vi "OM Setup.vi"() -> ()   [LabVIEW 2009]
uses:
  lib/Data Access Objects/Metadata/LBCB Number.ctl
  lib/Data Access Objects/Metadata/LBCB Settings.ctl
  lib/Data Access Objects/Metadata/LBCB Size.ctl
  lib/Data Access Objects/Metadata/LBCB Type.ctl
  lib/Data Access Objects/Application/Number Of LBCBs.ctl
  lib/Data Access Objects/Metadata/LBCB Location.ctl
  lib/Data Access Objects/Metadata/Actuator Matrix.ctl
  lib/Data Access Objects/Metadata/Actuator Point.ctl
  lib/Data Access Objects/Metadata/Cartesian Matrix.ctl
  lib/Data Access Objects/Metadata/Cartesian Point.ctl
  lib/Data Access Objects/Autobalance/Autobalance Control Parameters.ctl
  lib/Data Access Objects/Application/App Parameters.ctl
  lib/Data Access Objects/Application/Timing Parameters.ctl
  lib/Data Access Objects/Metadata/LBCB Position.ctl
  lib/MixedMode/Stiffness Matrix.ctl
  lib/Data Access Objects/Metadata/Cartesian Force Vector.ctl
  lib/Data Access Objects/Limits/Limit Boundary Parameters.ctl
  Popups/External Sensor Specs.ctl
  lib/Data Access Objects/Metadata/Actuator Channel Names.ctl
  lib/MixedMode/Ramp Time Input.ctl
  lib/MixedMode/Ramp Control.ctl
  lib/Data Access Objects/Application/Network Parameters.ctl
  lib/Data Access Objects/Mixed Mode/Force Control Parameters.ctl
  Popups/Update Actions.ctl
  lib/Data Access Objects/Metadata/Persistant DAO Actions.ctl
panel:
  in  "Rigid Connection":bool
  in  "LBCB Number Button":bool
  in  "Number of LBCBs":T1
  in  "Save":bool
  in  "Load":bool
  in  "OM Setup Page Tab":T2(tab)
  in  "Act Disp Bnd":T3 caption="Actuator Disp Limit \nBoundary Parameters"
  in  "Actuator Force Limits":T4
  in  "Actuator Stroke Limits":T4
  in  "Command Voltage Limit":T4
  in  "Act Force Bnd":T3 caption="Actuator Force Limit \nBoundary Parameters"
  in  "Cartesian Displacement":T6
  in  "Cartesian Force Limit":T6
  in  "Cart Force Bnd":T3 caption="Cartesian Force Limit \nBoundary Parameters"
  in  "Cart Trans Bnd":T3 caption="Cartesian Translation Limit \nBoundary Parameters"
  in  "Cart Rot Bnd":T3 caption="Cartesian Rotation Limit \nBoundary Parameters"
  in  "Cart Mmt Bnd":T3 caption="Cartesian Moment Limit \nBoundary Parameters"
  in  "Auto Balance Control":T8={"Number of Samples"=0, "Delay After Cmd"=0, "Maximum Command"=0.0, "1/4 Linear Range"=0.5}
  in  "Auto Balance Error Window":T5
  in  "I Gain":T5
  in  "P Gain":T5
  in  "NTCP Network":T9={"Port Number"=0, "Notification Name"="DataAvailableForTransmission", "Wait For Notification Timeout"=1000}
  in  "DAQ Link Network":T9={"Port Number"=0, "Notification Name"="DataAvailableForTransmission", "Wait For Notification Timeout"=1000}
  in  "Application Timing and Logging":T10
  in  "LBCB Position":T12={"Motion Center"=[0.0, 0.0, 0.0], "Transformation Matrix"=[[1.0, 0.0, 0.0, 0.0, 0.0, 0.0], [0.0, 1.0, 0.0, 0.0, 0.0, 0.0], [0.0, 0.0, 1.0, 0.0, 0.0, 0.0], [0.0, 0.0, 0.0, 1.0, 0.0, 0.0], [0.0, 0.0, 0.0, 0.0, 1.0, 0.0], [0.0, 0.0, 0.0, 0.0, 0.0, 1.0]]}
  in  "LBCB Settings":T13={"Size"=enum."1/5th-scale LBCB", "Type"=enum."Left Hand Type"}
  in  "Force Control Parameters":T16
  in  "Stiffness Limit":T6
  in  "Force Group Priorities":T7
  in  "Default Ramp Times":T17
  in  "Force Error Range":T19
  in  "Jacobian Gain":T7
  in  "Max Increment":T7
  in  "Stiffness Jacobian":T20=[[1000000.0, 0.0, 0.0, 0.0, 0.0, 0.0], [0.0, 1000000.0, 0.0, 0.0, 0.0, 0.0], [0.0, 0.0, 1000000.0, 0.0, 0.0, 0.0], [0.0, 0.0, 0.0, 1000000.0, 0.0, 0.0], [0.0, 0.0, 0.0, 0.0, 1000000.0, 0.0], [0.0, 0.0, 0.0, 0.0, 0.0, 1000000.0]]
  in  "Servo Error Offset":T5
  in  "LVDT  Offset":T5
  in  "Load Cell  Offset":T5
  in  "Load Cell Sensitivity":T5
  in  "Command Sensitivity":T5
  in  "LVDT Sensitivity":T5
  in  "Command Channels":T21
  in  "LVDT Channels":T21
  in  "Load Cell Channels":T21
  in  "Servo Error  Channels":T21
  in  "External Sensor Specs":T22[](array[typedef])
  in  "OM  Location":T23
  in  "Ok":bool
  in  "LBCB Number":T24
  # "(Volts)"
  # "Interval is in Seconds\nRate is in Samples per Second"
  # "(inch)"
  # "X"
  # "(inch)"
  # "Y"
  # "(inch)"
  # "Z"
  # "Xglobal = T*Xlocal"
  # "DAQMx Global Channel"
  # "Display Name"
  # "Sensiitivity"
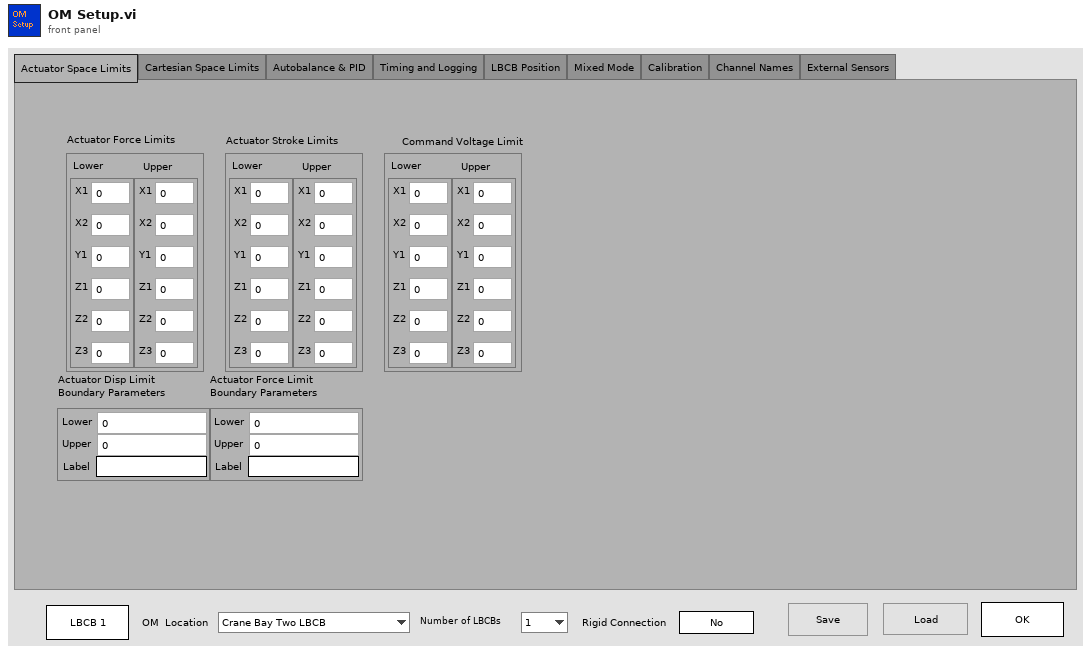
[diagram p1: front panel]
types:
  T1 = typedef "Number Of LBCBs.ctl" = enum16{"1", "2"}
  T2 = enum32{"Actuator Space Limits", "Cartesian Space Limits", "Autobalance & PID", "Timing and Logging", "LBCB Position", "Mixed Mode", "Calibration", "Channel Names", "External Sensors"}
  T3 = typedef "Limit Boundary Parameters.ctl" = cluster{"Lower":dbl, "Upper":dbl, "Label":string}
  T4 = typedef "Actuator Matrix.ctl" = cluster{"Lower":T5, "Upper":T5}
  T5 = typedef "Actuator Point.ctl" = cluster{"X1":dbl, "X2":dbl, "Y1":dbl, "Z1":dbl, "Z2":dbl, "Z3":dbl}
  T6 = typedef "Cartesian Matrix.ctl" = cluster{"Lower":T7, "Upper":T7}
  T7 = typedef "Cartesian Point.ctl" = cluster{"Dx":dbl, "Dy":dbl, "Dz":dbl, "Rx":dbl, "Ry":dbl, "Rz":dbl}
  T8 = typedef "Autobalance Control Parameters.ctl" = cluster{"Number of Samples":i32, "Delay After Cmd":i32, "Maximum Command":dbl, "1/4 Linear Range":dbl}
  T9 = typedef "Network Parameters.ctl" = cluster{"Port Number":u16, "Notification Name":string, "Wait For Notification Timeout":i32}
  T10 = typedef "App Parameters.ctl" = cluster{"Monitor Loop":T11, "Ramp Time":T11, "Log Loop":T11, "TCP to DAQ":T11, "Logging Directory":path, "Log File Size (MBytes)":i64, "Volt Logging Loop":T11}
  T11 = typedef "Timing Parameters.ctl" = cluster{"Interval":dbl, "Rate ":dbl}
  T12 = typedef "LBCB Position.ctl" = cluster{"Motion Center":dbl[], "Transformation Matrix":dbl[][]}
  T13 = typedef "LBCB Settings.ctl" = cluster{"Size":T14, "Type":T15}
  T14 = typedef "LBCB Size.ctl" = enum16{"1/5th-scale LBCB", "Full-scale LBCB", "Portable LBCB"}
  T15 = typedef "LBCB Type.ctl" = enum16{"Right Hand Type", "Left Hand Type"}
  T16 = typedef "Force Control Parameters.ctl" = cluster{"Use Force Error Range Ratios":bool, "Use Group Priorities":bool, "Multi Command Update":bool, "Use Tru Mixed Mode":bool}
  T17 = typedef "Ramp Time Input.ctl" = cluster{"Directional":T18, "Iterative":T18}
  T18 = typedef "Ramp Control.ctl" = cluster{"Ramp":dbl, "Stabilize":dbl, "Hold":dbl}
  T19 = typedef "Cartesian Force Vector.ctl" = cluster{"Fx":dbl, "Fy":dbl, "Fz":dbl, "Mx":dbl, "My":dbl, "Mz":dbl}
  T20 = typedef "Stiffness Matrix.ctl" = dbl[][]
  T21 = typedef "Actuator Channel Names.ctl" = cluster{"X1":refnum<k21>, "X2":refnum<k21>, "Y1":refnum<k21>, "Z1":refnum<k21>, "Z2":refnum<k21>, "Z3":refnum<k21>}
  T22 = typedef "External Sensor Specs.ctl" = cluster{"DAQmx Global Channel":refnum<k21>, "Display Name":string, "Sensitivity":dbl}
  T23 = typedef "LBCB Location.ctl" = enum16{"Crane Bay Two LBCB", "Crane Bay One LBCB", "5th Scale Two LBCB", "5th Scale One LBCB", "Portable LBCB"}
  T24 = typedef "LBCB Number.ctl" = enum16{"LBCB1", "LBCB2"}
  T25 = typedef "Update Actions.ctl" = enum16{"Update", "Exit"}
  T26 = typedef "Persistant DAO Actions.ctl" = enum16{"Init", "Get", "Set", "Load", "Save"}
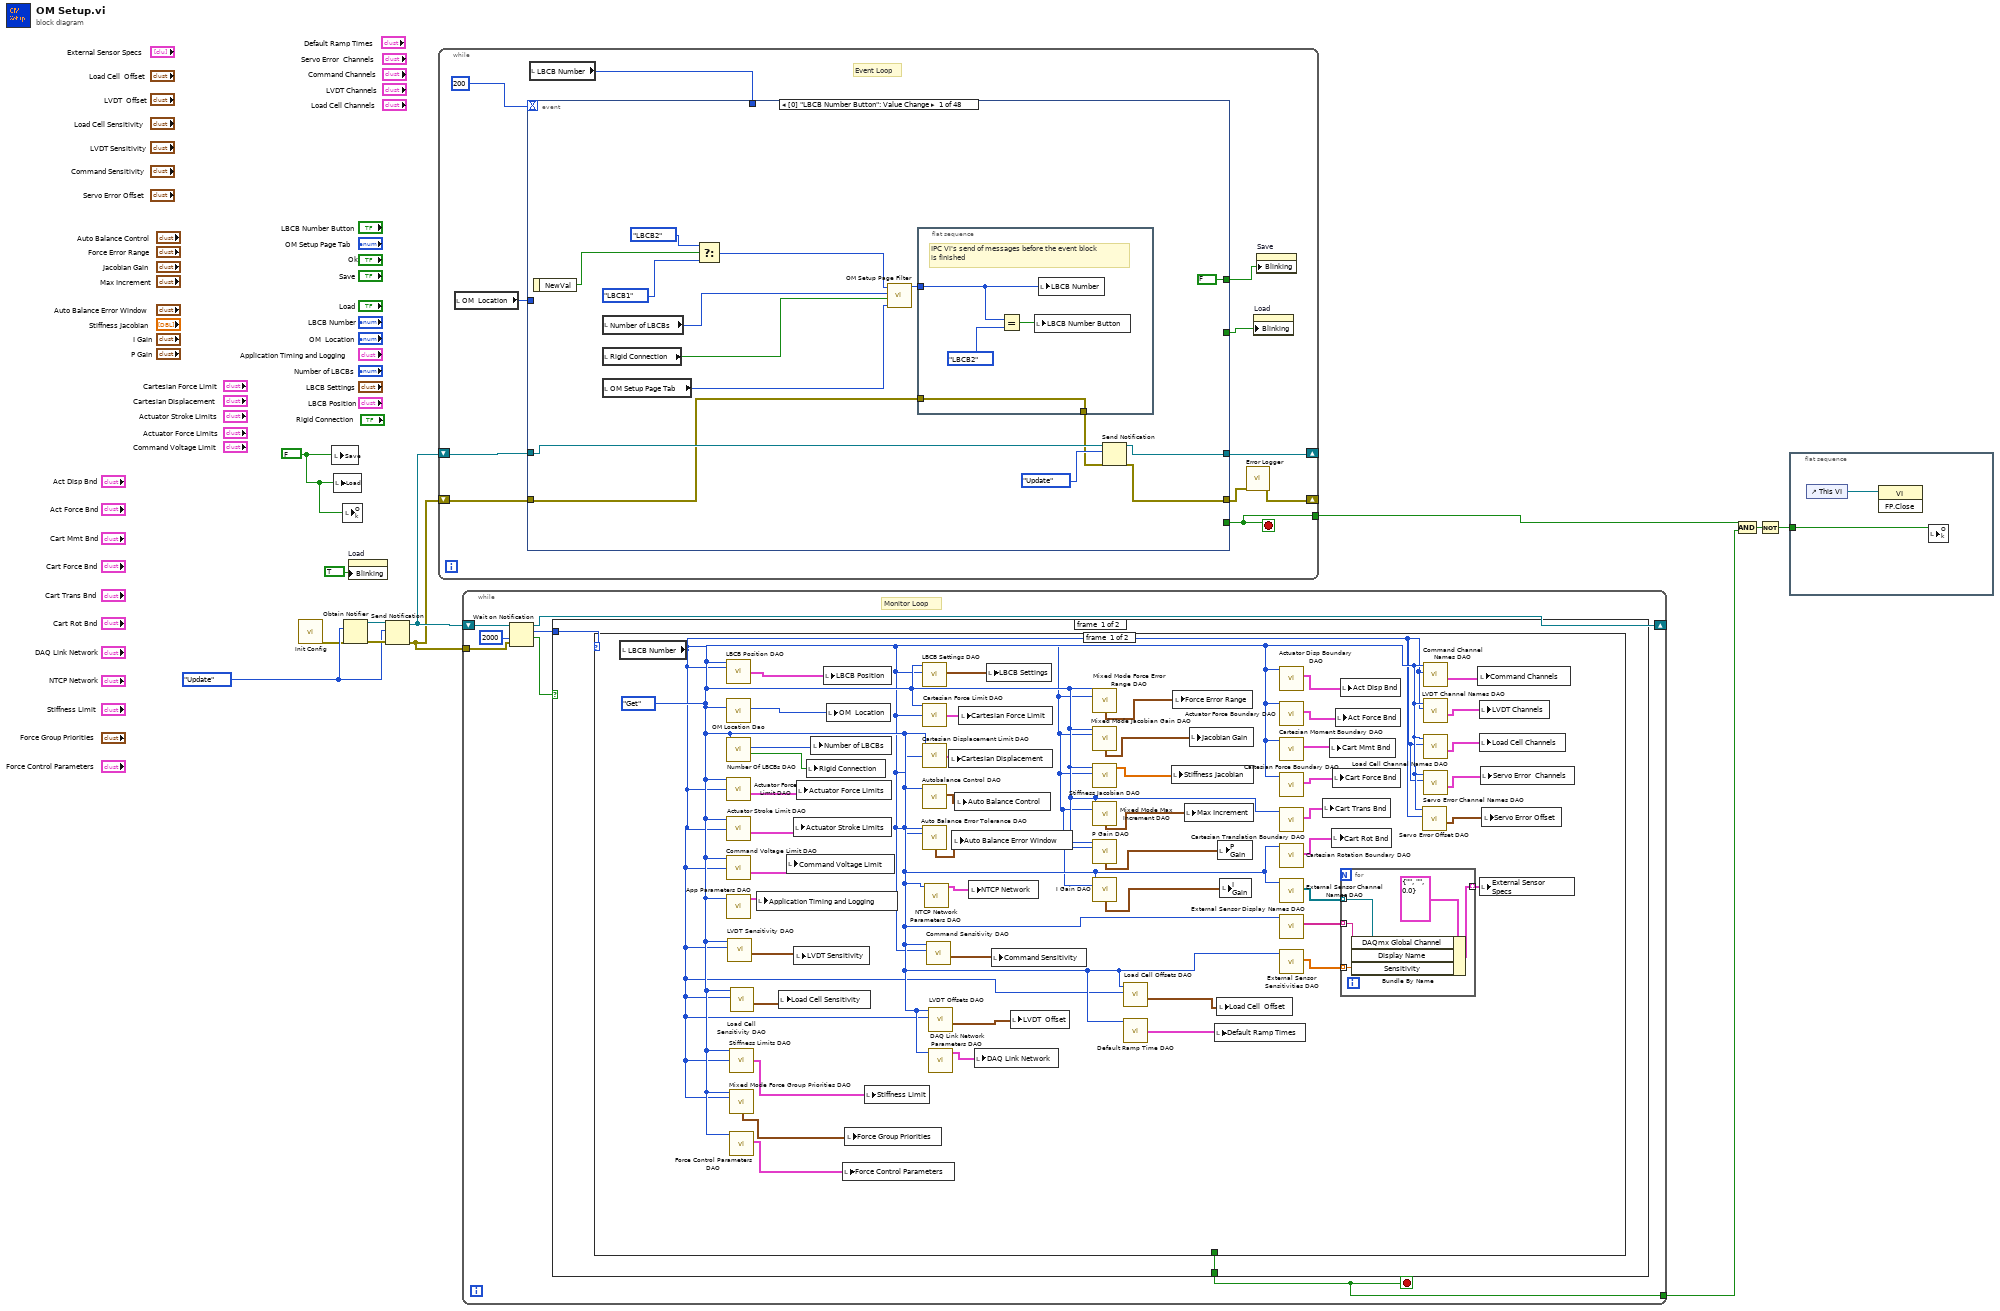
[diagram p0: block diagram]
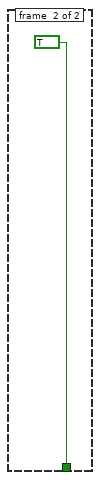
[diagram p2: hidden frame]
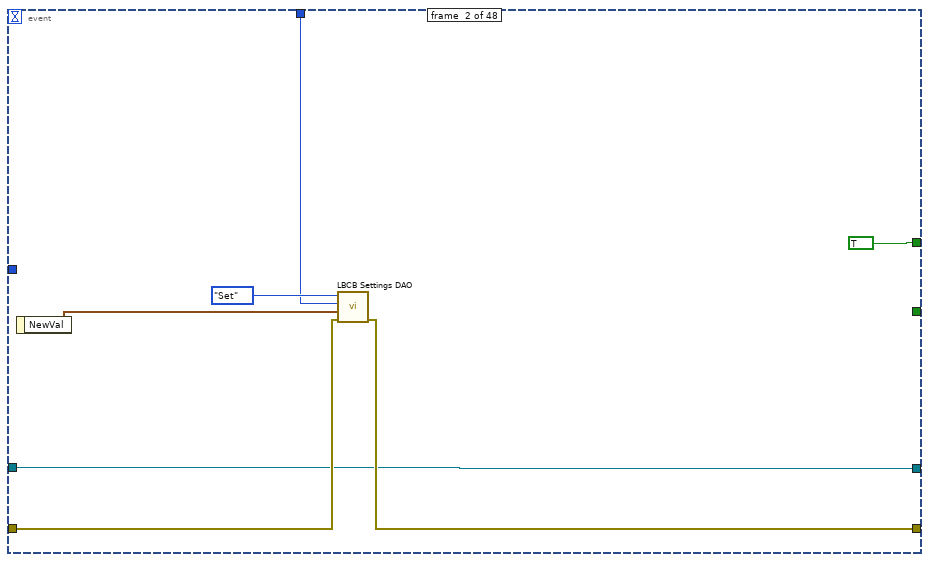
[diagram p4: hidden frame]
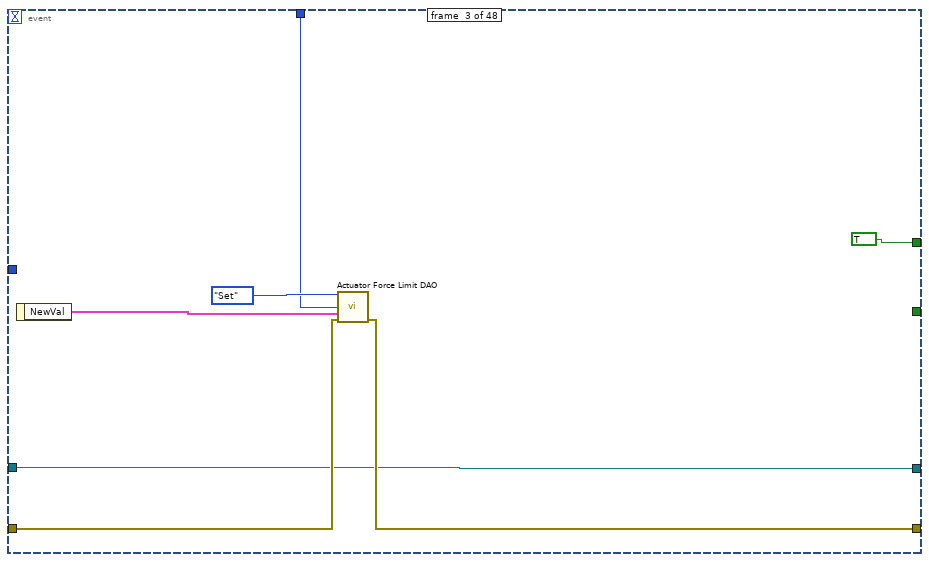
[diagram p5: hidden frame]
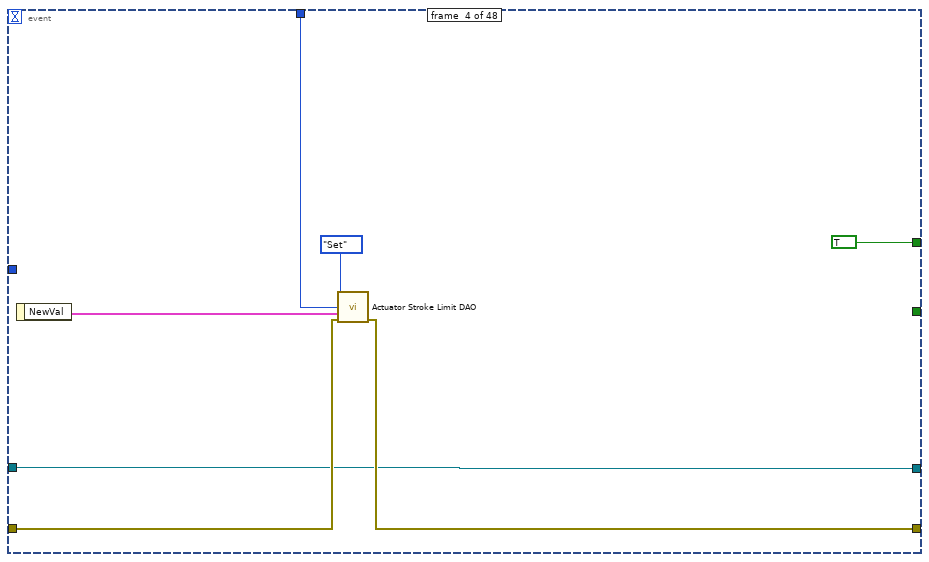
[diagram p6: hidden frame]
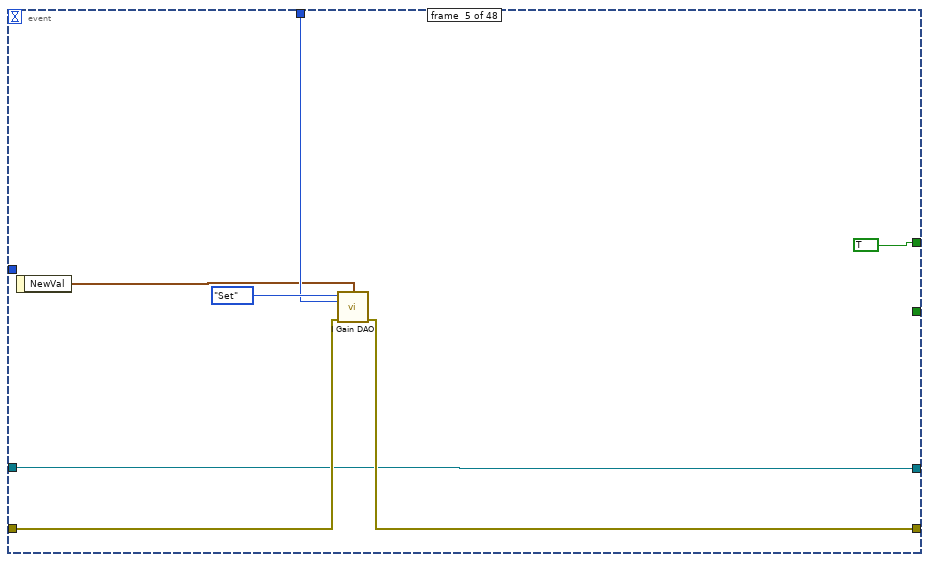
[diagram p7: hidden frame]
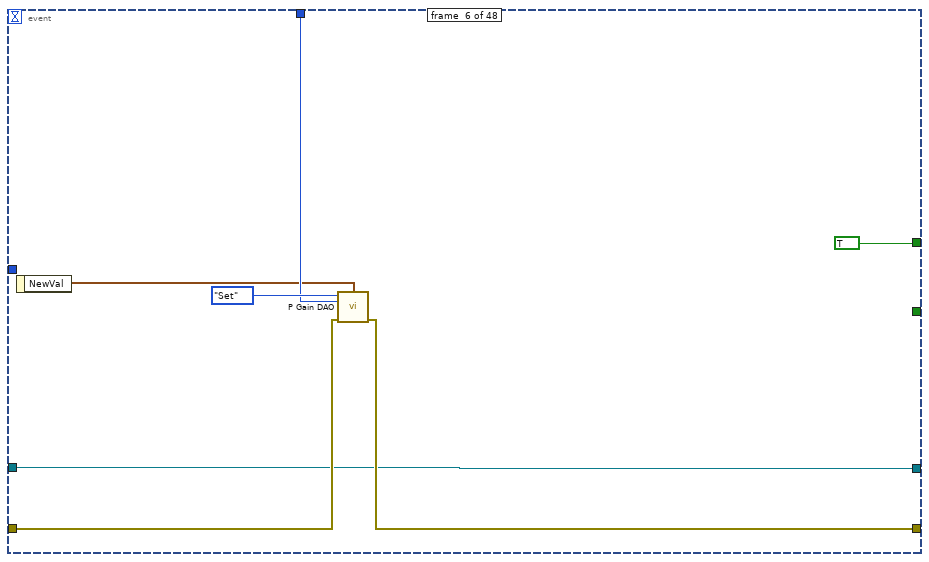
[diagram p8: hidden frame]
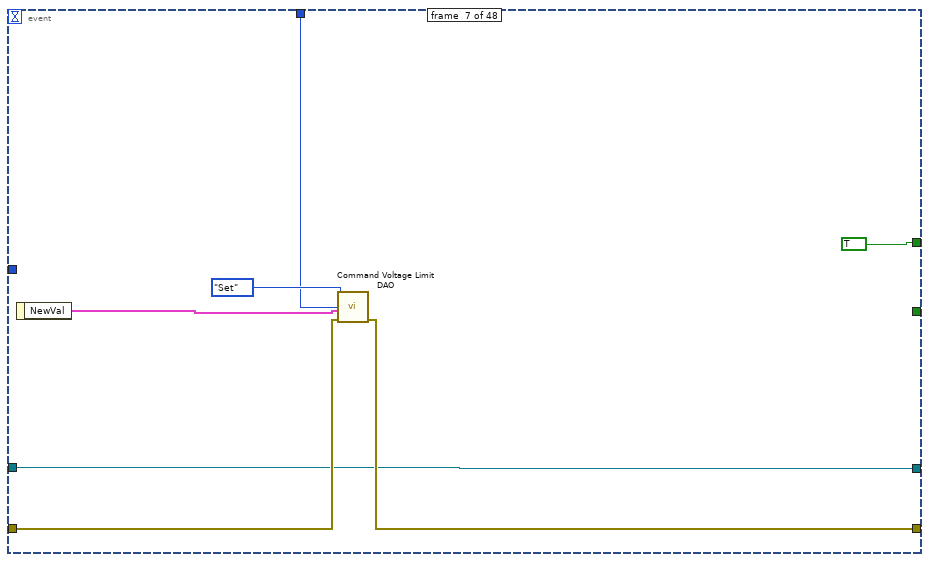
[diagram p9: hidden frame]
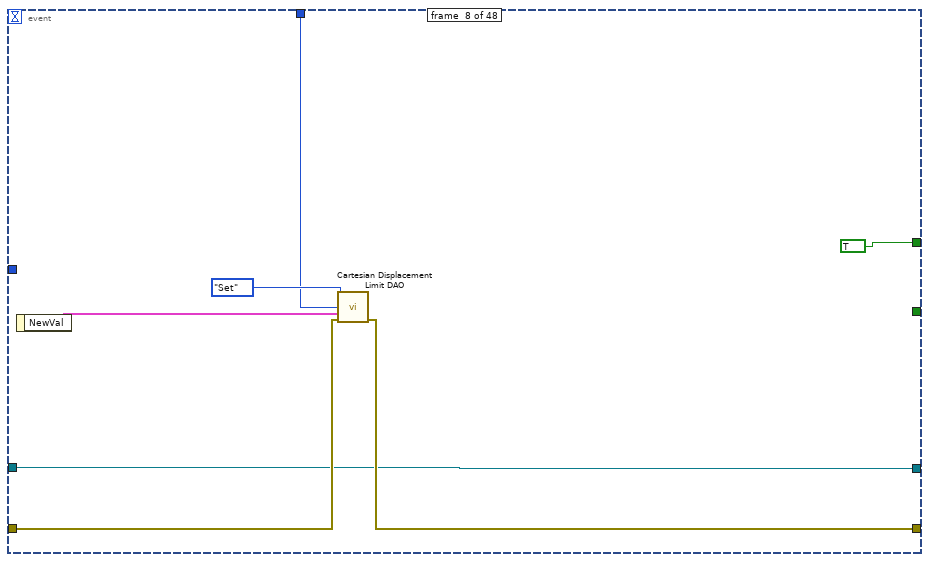
[diagram p10: hidden frame]
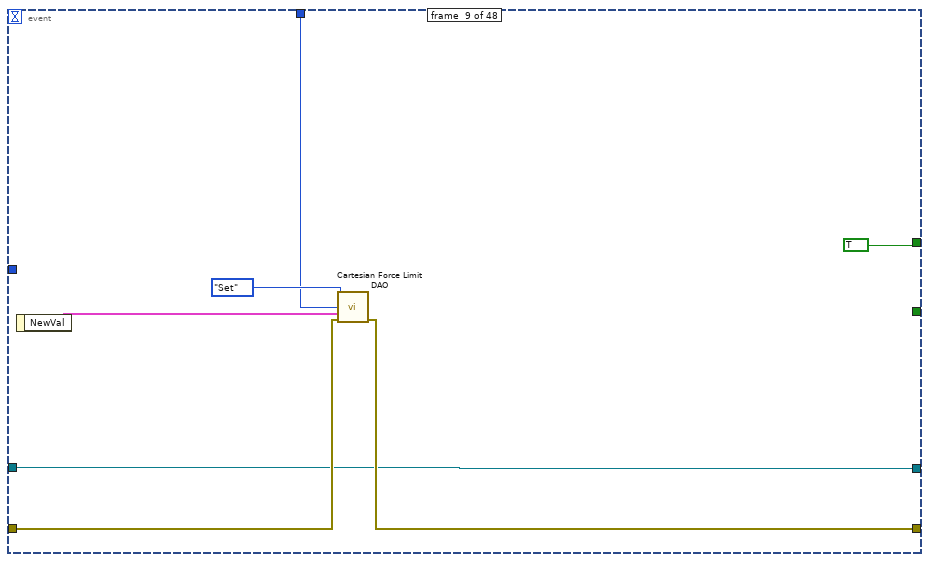
[diagram p11: hidden frame]
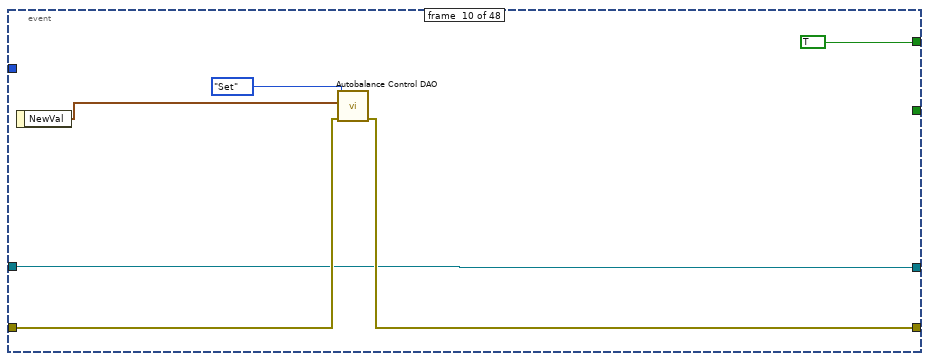
[diagram p12: hidden frame]
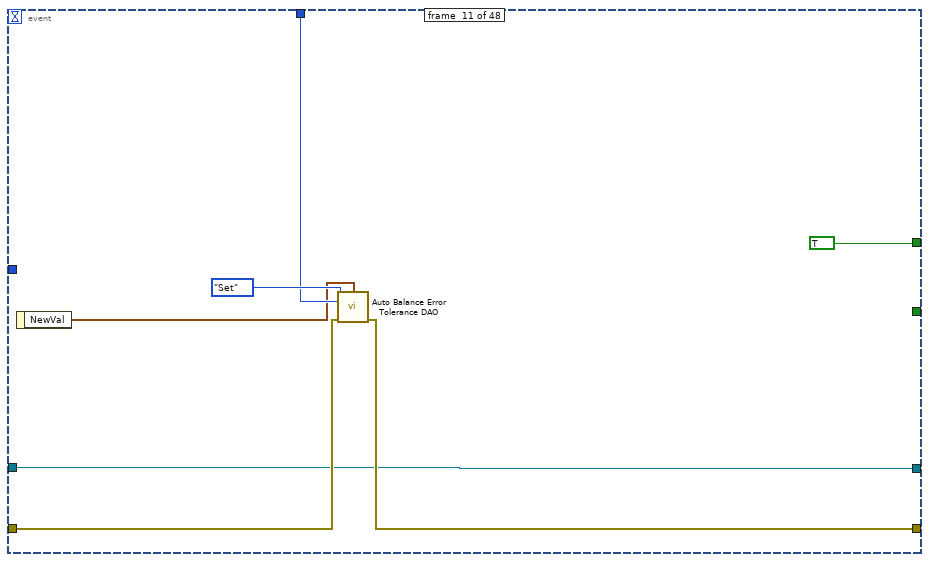
[diagram p13: hidden frame]
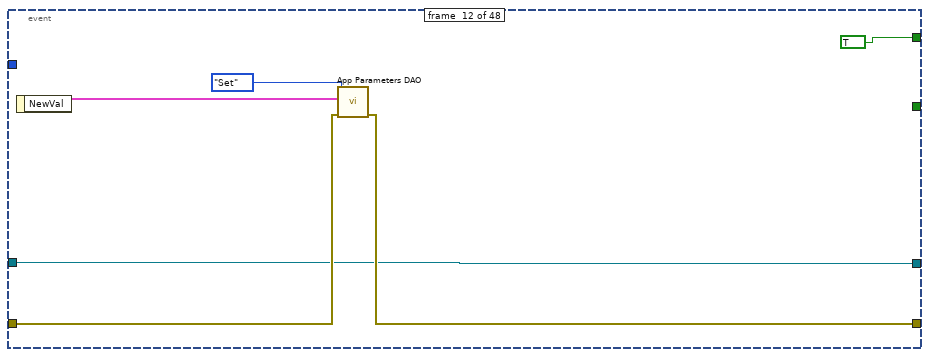
[diagram p14: hidden frame]
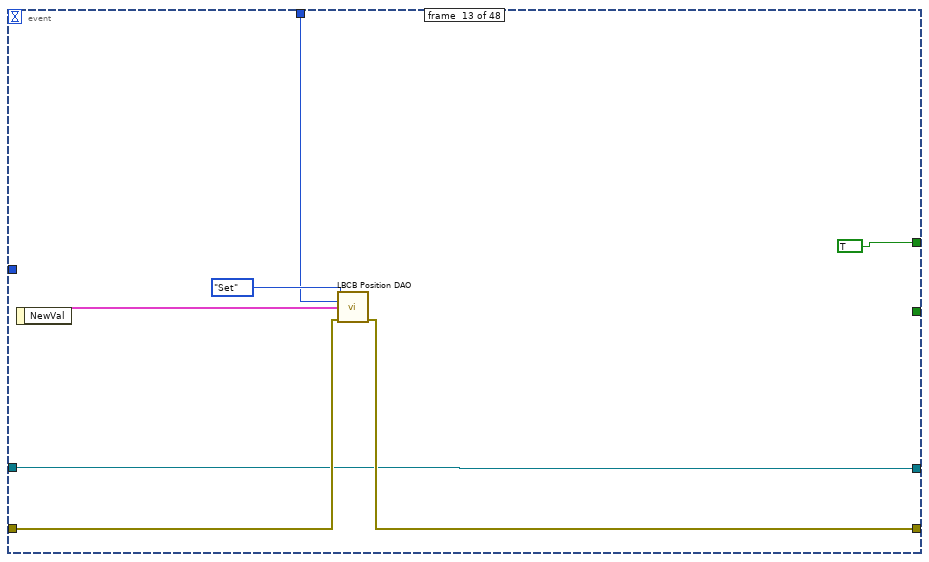
[diagram p15: hidden frame]
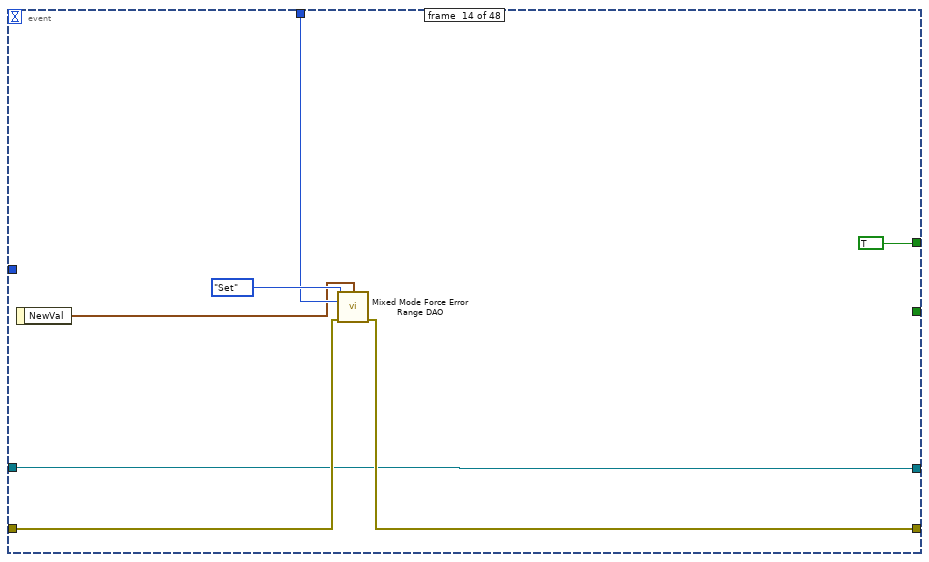
[diagram p16: hidden frame]
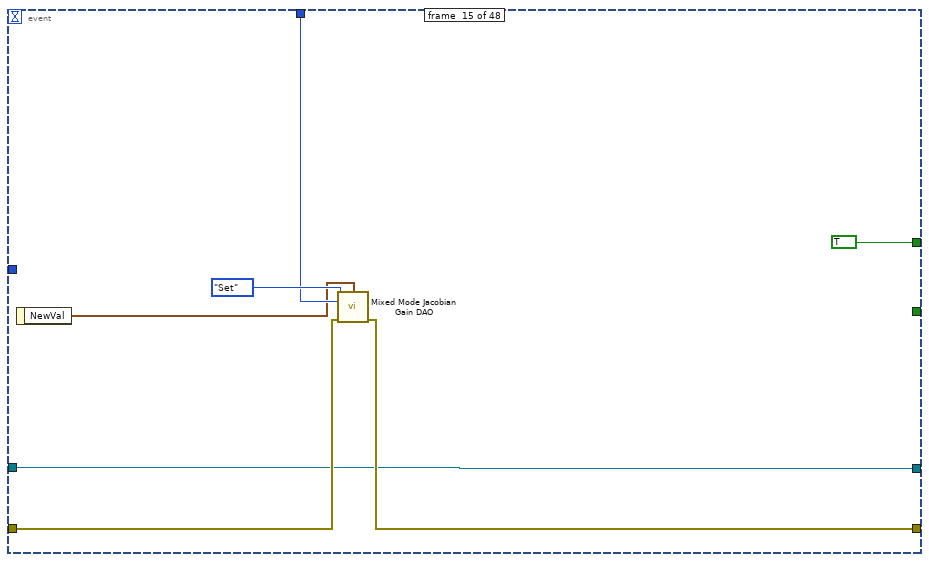
[diagram p17: hidden frame]
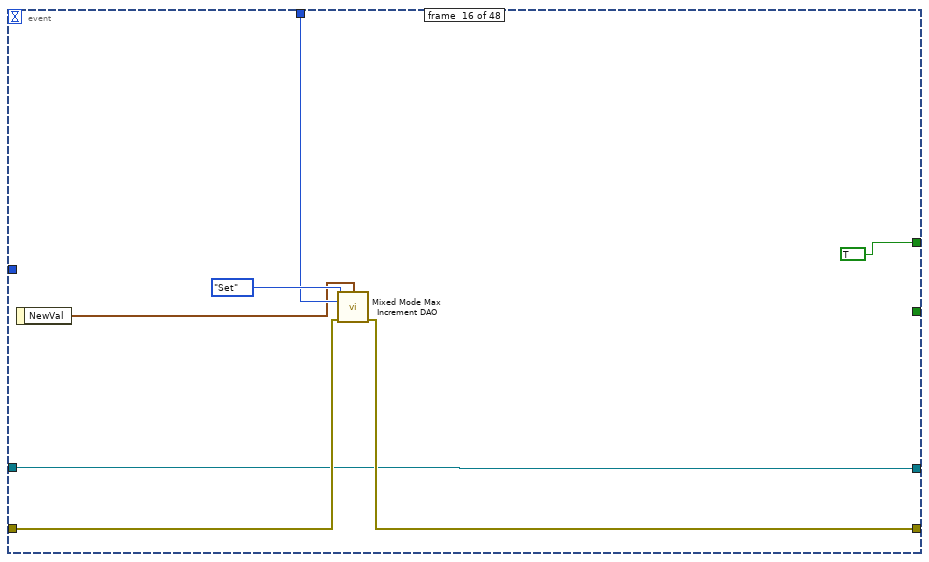
[diagram p18: hidden frame]
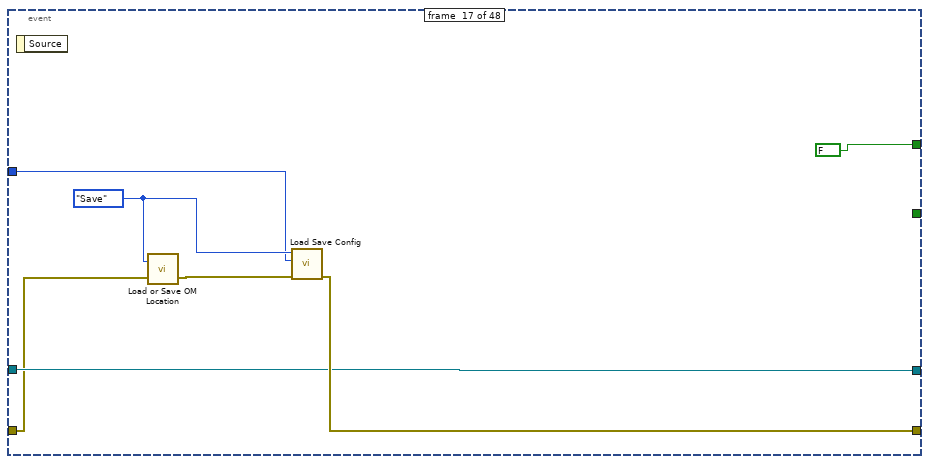
[diagram p19: hidden frame]
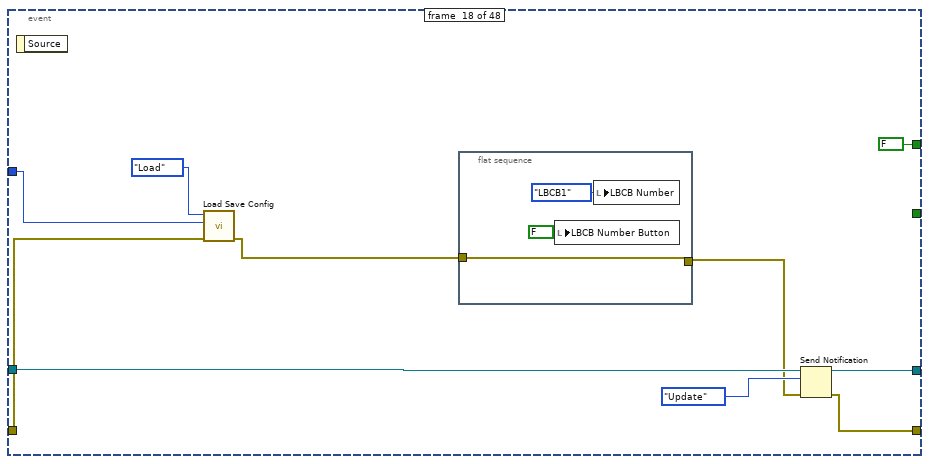
[diagram p20: hidden frame]
diagram:
  w5 = FALSE ("Save")
  w10 = Update_Actions."Update" ("Update Actions")
  n1 = call "Init Config.vi"() -> ("error out"=w7:errorcluster)  [unwired: 1 in, 10 out]
  n2 = local write "Save"(w5) -> ()
  n3 = local write "Load"(w5) -> ()
  n4 = local write "Ok"(w5) -> ()
  n5 = Obtain Notifier(notification data type=w10, error in (no error)=w7) -> (notifier out=w12:refnum<notifier>, error out=w11:errorcluster)  [unwired: 1 in, 2 out]
  n6 = property on="Load" class="Bool (strict)"("Blinking"=TRUE) -> ()  [unwired: 2 in, 2 out]
  n7 = Send Notification(notification=w10, notifier=w12, error in (no error)=w11) -> (notifier out=w9:refnum<notifier>, error out=w8:errorcluster)
  n8 = while {
    shift-right: [w21] -> _
    shift-left: w8 -> [w23]
    shift-right: [w19] -> _
    shift-left: w9 -> [w20]
    tunnel: [w13] -> w4
    stop <- w13 stop-if-true
    # "Event Loop"
    n9 = local read "OM  Location"() -> (w14:T23)
    n10 = local read "LBCB Number"() -> (w18:T24)
    n11 = event shown="[0] \"LBCB Number Button\": Value Change" {
      selector: _ -> [_ _ _ _ _ _ _ _ _ _ _ _ _ _ _ _ _ _ _ _ _ _ _ _ _ _ _ _ _ _ _ _ _ _ _ _ _ _ _ _ _ _ _ _ _ _ _ _]
      dyn-events: _ -> [_ _ _ _ _ _ _ _ _ _ _ _ _ _ _ _ _ _ _ _ _ _ _ _ _ _ _ _ _ _ _ _ _ _ _ _ _ _ _ _ _ _ _ _ _ _ _ _]
      timeout: 200 -> [_ _ _ _ _ _ _ _ _ _ _ _ _ _ _ _ _ _ _ _ _ _ _ _ _ _ _ _ _ _ _ _ _ _ _ _ _ _ _ _ _ _ _ _ _ _ _ _]
      tunnel: w23 -> [w25 w46 w54 w61 w68 w75 w82 w89 w96 w103 w109 w116 w122 w129 w136 w143 w148 w156 w176 w190 w202 w214 w222 w228 w234 w240 w246 w252 w259 w264 w273 w279 w286 w293 w296 w321 w328 w335 w342 w349 w355 w361 w367 w373 w380 w387 w396 w417]
      tunnel: [w38 w45 w53 w60 w67 w74 w81 w88 w95 w102 w108 w115 w121 w128 w135 w142 w152 w159 w170 w190 w201 w214 w221 w227 w233 w239 w245 w251 w258 w263 w274 w278 w285 w292 w296 w322 w329 w336 w343 w350 w354 w360 w366 w372 w379 w386 w395 w416] -> w22
      tunnel: w20 -> [w37 w44 w52 w59 w66 w73 w80 w87 w94 w101 w107 w114 w120 w127 w134 w141 w151 w162 w173 w191 w203 w213 w220 w226 w232 w238 w244 w250 w257 w267 w269 w276 w282 w290 w304 w317 w325 w332 w339 w346 w353 w359 w365 w371 w378 w385 w397 w415]
      tunnel: [w36 w44 w52 w59 w66 w73 w80 w87 w94 w101 w107 w114 w120 w127 w134 w141 w151 w160 w172 w191 w200 w213 w220 w226 w232 w238 w244 w250 w257 w267 w269 w276 w282 w290 w304 w317 w325 w332 w339 w346 w353 w359 w365 w371 w378 w385 w394 w414] -> w19
      tunnel: w18 -> [_ w47 w55 w62 w69 w76 w83 w90 w97 _ w110 _ w123 w130 w137 w144 _ _ _ _ _ _ _ _ _ _ _ _ w254 w265 w271 w281 w288 w295 _ w319 w326 w333 w340 w347 _ _ _ w374 w381 _ _ w408]
      tunnel: [_ _ _ _ _ _ _ _ _ _ _ _ _ _ _ _ _ _ TRUE _ _ _ _ _ _ _ _ _ _ _ _ _ _ _ _ _ _ _ _ _ _ _ _ _ _ _ _ _] -> w13
      tunnel: [FALSE ("Blinking") TRUE ("Blinking") TRUE ("Blinking") TRUE ("Blinking") TRUE ("Blinking") TRUE ("Blinking") TRUE ("Blinking") TRUE ("Blinking") TRUE ("Blinking") TRUE ("Blinking") TRUE ("Blinking") TRUE ("Blinking") TRUE ("Blinking") TRUE ("Blinking") TRUE ("Blinking") TRUE ("Blinking") FALSE ("Blinking") FALSE ("Blinking") FALSE ("Blinking") FALSE ("Blinking") TRUE ("Blinking") w216 TRUE ("Blinking") TRUE ("Blinking") TRUE ("Blinking") TRUE ("Blinking") TRUE ("Blinking") TRUE ("Blinking") TRUE ("Blinking") TRUE ("Blinking") TRUE ("Blinking") TRUE ("Blinking") TRUE ("Blinking") TRUE ("Blinking") TRUE ("Blinking") TRUE ("Blinking") TRUE ("Blinking") TRUE ("Blinking") TRUE ("Blinking") TRUE ("Blinking") TRUE ("Blinking") TRUE ("Blinking") TRUE ("Blinking") TRUE ("Blinking") TRUE ("Blinking") TRUE ("Blinking") TRUE ("Blinking") FALSE ("Blinking")] -> w17
      tunnel: [_ _ _ _ _ _ _ _ _ _ _ _ _ _ _ _ _ _ _ TRUE ("Blinking") _ w215 _ _ _ _ _ _ _ _ _ _ _ _ _ _ _ _ _ _ _ _ _ _ _ _ _ _] -> w16
      tunnel: w14 -> [_ _ _ _ _ _ _ _ _ _ _ _ _ _ _ _ w146 w153 w166 _ _ _ _ _ _ _ _ _ _ _ _ _ _ _ _ _ _ _ _ _ _ _ _ _ _ _ _ _]
      event #0 {
        n12 = event-data() -> ("NewVal"=w31:bool)  [unwired: 1 out]
        n13 = local read "Number of LBCBs"() -> (w29:T1)
        n14 = local read "Rigid Connection"() -> (w28:bool)
        n15 = local read "OM Setup Page Tab"() -> (w27:T2)
        n16 = Select(t=LBCB_Number."LBCB2", s=w31, f=LBCB_Number."LBCB1" ("LBCB Number")) -> (s? t:f=w30:T24)
        n17 = call "OM Setup Page Filter.vi"("OM Setup Page"=w27, "Rigid Connection In"=w28, "Number of\nLBCBs In"=w29, "LBCB Number In"=w30) -> ("LBCB Number Out"=w26:T24)  [unwired: 7 in]
        n18 = flat-sequence {
          tunnel: w26 -> [w41]
          tunnel: w25 -> [w39]
          tunnel: [w39] -> w24
          frame #0 {
            # "IPC Vi's send of messages before the event block\nis finished"
            n19 = Equal?(x=w41, y=LBCB_Number."LBCB2") -> (x = y?=w42:bool)
            n20 = local write "LBCB Number Button"(w42) -> ()
            n21 = local write "LBCB Number"(w41) -> ()
          }
        }
        n22 = Send Notification(notification=Update_Actions."Update", notifier=w37, error in (no error)=w24) -> (notifier out=w36:refnum<notifier>, error out=w38:errorcluster)
      }
      event #1 {
        n23 = event-data() -> ("NewVal"=w49:T13)  [unwired: 1 out]
        n24 = call "LBCB Settings DAO.vi"("error in (no error)"=w46, "LBCB Setting In"=w49, "LBCB Number"=w47, "Actions"=Persistant_DAO_Actions."Set") -> ("error out"=w45:errorcluster)  [unwired: 1 in, 6 out]
      }
      event #2 {
        n25 = event-data() -> ("NewVal"=w51:T4)  [unwired: 1 out]
        n26 = call "Actuator Force Limit DAO.vi"("Actuator Force Limit Actions"=Persistant_DAO_Actions."Set" ("Actions"), "ID"=w55, "Actuator Force Limits  Input"=w51, "error in (no error)"=w54) -> ("error out"=w53:errorcluster)  [unwired: 1 in, 10 out]
      }
      event #3 {
        n27 = event-data() -> ("NewVal"=w58:T4)  [unwired: 1 out]
        n28 = call "Actuator Stroke Limit DAO.vi"("Actuator Stroke Limit Actions"=Persistant_DAO_Actions."Set" ("Actions"), "ID"=w62, "Actuator Stroke Limits In"=w58, "error in (no error)"=w61) -> ("error out"=w60:errorcluster)  [unwired: 1 in, 10 out]
      }
      event #4 {
        n29 = event-data() -> ("NewVal"=w65:T5)  [unwired: 1 out]
        n30 = call "I Gain DAO.vi"("I Gain Actions"=Persistant_DAO_Actions."Set" ("Actions"), "I Gain In"=w65, "LBCB Number"=w69, "error in (no error)"=w68) -> ("error out"=w67:errorcluster)  [unwired: 2 in, 9 out]
      }
      event #5 {
        n31 = event-data() -> ("NewVal"=w72:T5)  [unwired: 1 out]
        n32 = call "P Gain DAO.vi"("P Gain Actions"=Persistant_DAO_Actions."Set" ("Actions"), "P Gain In"=w72, "LBCB Number"=w76, "error in (no error)"=w75) -> ("error out"=w74:errorcluster)  [unwired: 1 in, 10 out]
      }
      event #6 {
        n33 = event-data() -> ("NewVal"=w79:T4)  [unwired: 1 out]
        n34 = call "Command Voltage Limit DAO.vi"("Actuator Stroke Limit Actions"=Persistant_DAO_Actions."Set" ("Actions"), "ID"=w83, "Command Voltage Limit In"=w79, "error in (no error)"=w82) -> ("error out"=w81:errorcluster)  [unwired: 2 in, 9 out]
      }
      event #7 {
        n35 = event-data() -> ("NewVal"=w86:T6)  [unwired: 1 out]
        n36 = call "Cartesian Displacement Limit DAO.vi"("Cartesian Displacement Limit Actions"=Persistant_DAO_Actions."Set" ("Actions"), "ID"=w90, "Cartesian Displacement In"=w86, "error in (no error)"=w89) -> ("error out"=w88:errorcluster)  [unwired: 1 in, 10 out]
      }
      event #8 {
        n37 = event-data() -> ("NewVal"=w93:T6)  [unwired: 1 out]
        n38 = call "Cartesian Force Limit DAO.vi"("Cartesian Force Limit Actions"=Persistant_DAO_Actions."Set" ("Actions"), "ID"=w97, "Cartesian Force Limit In"=w93, "error in (no error)"=w96) -> ("error out"=w95:errorcluster)  [unwired: 1 in, 10 out]
      }
      event #9 {
        n39 = event-data() -> ("NewVal"=w99:T8)  [unwired: 1 out]
        n40 = call "Autobalance Control DAO.vi"("error in (no error)"=w103, "Autobalance Control In"=w99, "Persistent DAO Actions"=Persistant_DAO_Actions."Set" ("Actions")) -> ("error out"=w102:errorcluster)  [unwired: 2 in, 6 out]
      }
      event #10 {
        n41 = event-data() -> ("NewVal"=w106:T5)  [unwired: 1 out]
        n42 = call "Auto Balance Error Tolerance DAO.vi"("Auto Balance Increment Actions"=Persistant_DAO_Actions."Set" ("Actions"), "Auto Balance Error In"=w106, "LBCB Number"=w110, "error in (no error)"=w109) -> ("error out"=w108:errorcluster)  [unwired: 1 in, 10 out]
      }
      event #11 {
        n43 = event-data() -> ("NewVal"=w113:T10)  [unwired: 1 out]
        n44 = call "App Parameters DAO.vi"("error in (no error)"=w116, "Application Timing and Logging In"=w113, "Actions"=Persistant_DAO_Actions."Set") -> ("error out"=w115:errorcluster)  [unwired: 1 in, 7 out]
      }
      event #12 {
        n45 = event-data() -> ("NewVal"=w119:T12)  [unwired: 1 out]
        n46 = call "LBCB Position DAO.vi"("LBCB Settings Actions"=Persistant_DAO_Actions."Set" ("Actions"), "LBCB Number"=w123, "LBCB Position In"=w119, "error in (no error)"=w122) -> ("error out"=w121:errorcluster)  [unwired: 1 in, 10 out]
      }
      event #13 {
        n47 = event-data() -> ("NewVal"=w126:T19)  [unwired: 1 out]
        n48 = call "Mixed Mode Force Error Range DAO.vi"("Force Error Range Actions"=Persistant_DAO_Actions."Set" ("Actions"), "Force Error Range In"=w126, "LBCB Number"=w130, "error in (no error)"=w129) -> ("error out"=w128:errorcluster)  [unwired: 2 in, 9 out]
      }
      event #14 {
        n49 = event-data() -> ("NewVal"=w133:T7)  [unwired: 1 out]
        n50 = call "Mixed Mode Jacobian Gain DAO.vi"("Jacobian Gain Actions"=Persistant_DAO_Actions."Set" ("Actions"), "Jacobian Gain In"=w133, "LBCB Number"=w137, "error in (no error)"=w136) -> ("error out"=w135:errorcluster)  [unwired: 1 in, 10 out]
      }
      event #15 {
        n51 = event-data() -> ("NewVal"=w140:T7)  [unwired: 1 out]
        n52 = call "Mixed Mode Max Increment DAO.vi"("Max Increment Actions"=Persistant_DAO_Actions."Set" ("Actions"), "Max Increment In"=w140, "LBCB Number"=w144, "error in (no error)"=w143) -> ("error out"=w142:errorcluster)  [unwired: 1 in, 10 out]
      }
      event #16 {
        w149 = Persistant_DAO_Actions."Save" ("Actions")
        n53 = event-data() -> ()  [unwired: 2 out]
        n54 = call "Load or Save OM Location.vi"("error in (no error)"=w148, "Action"=w149) -> ("error out"=w150:errorcluster)  [unwired: 1 out]
        n55 = call "Load Save Config.vi"("error in (no error)"=w150, "OM  Location"=w146, "Actions"=w149) -> ("error out"=w152:errorcluster)  [unwired: 8 out]
      }
      event #17 {
        n56 = event-data() -> ()  [unwired: 2 out]
        n57 = call "Load Save Config.vi"("error in (no error)"=w156, "OM  Location"=w153, "Actions"=Persistant_DAO_Actions."Load") -> ("error out"=w155:errorcluster)  [unwired: 8 out]
        n58 = flat-sequence {
          tunnel: w155 -> [w165]
          tunnel: [w165] -> w154
          frame #0 {
            n59 = local write "LBCB Number Button"(FALSE ("LBCB Number Button")) -> ()
            n60 = local write "LBCB Number"(LBCB_Number."LBCB1" ("LBCB Number")) -> ()
          }
        }
        n61 = Send Notification(notification=Update_Actions."Update", notifier=w162, error in (no error)=w154) -> (notifier out=w160:refnum<notifier>, error out=w159:errorcluster)
      }
      event #18 {
        n62 = event-data() -> ()  [unwired: 2 out]
        n63 = property on="Save" class="Bool (strict)"() -> ("Blinking"=w167:bool)  [unwired: 2 in, 2 out]
        n64 = case shown="False" w167 {
          selector: w167 -> [w177 _]
          tunnel: [w177 w178] -> w175
          frame #0 {
          }
          frame #1 {
            n65 = Two Button Dialog(message="Do you want to save\nbefore loading the \nnew settings", 1:"No" ("F button name (\"Cancel\")"), 2:"Yes" ("T button name (\"OK\")")) -> (T button?=w178:bool)
          }
        }
        n66 = case shown="True" w175 {
          tunnel: [w182 w187] -> w171
          tunnel: w176 -> [w182 w184]
          tunnel: w166 -> [_ w183]
          frame #0 {
          }
          frame #1 {
            w185 = Persistant_DAO_Actions."Save" ("Actions")
            n67 = call "Load or Save OM Location.vi"("error in (no error)"=w184, "Action"=w185) -> ("error out"=w186:errorcluster)  [unwired: 1 out]
            n68 = call "Load Save Config.vi"("error in (no error)"=w186, "OM  Location"=w183, "Actions"=w185) -> ("error out"=w187:errorcluster)  [unwired: 8 out]
          }
        }
        n69 = Send Notification(notification=Update_Actions."Exit", notifier=w173, error in (no error)=w171) -> (notifier out=w172:refnum<notifier>, error out=w170:errorcluster)
      }
      event #19 {
        n70 = event-data() -> ("NewVal"=w192:T23)  [unwired: 1 out]
        n71 = call "OM Location Dao.vi"("LBCB  Location In"=w192, "Actions"=Persistant_DAO_Actions."Set") -> ()  [unwired: 2 in, 8 out]
      }
      event #20 {
        n72 = event-data() -> ("NewVal"=w197:T1)  [unwired: 1 out]
        n73 = local read "Rigid Connection"() -> (w196:bool)
        n74 = Select(t=Number_Of_LBCBs."2", s=w196, f=w197) -> (s? t:f=w194:T1)
        n75 = case shown="\"2\"" w194 {
          tunnel: w203 -> [w208 w212]
          tunnel: w202 -> [w207 w211]
          tunnel: [w206 w211] -> w201
          tunnel: [w205 w212] -> w200
          frame #0 {
            n76 = local write "LBCB Number Button"(FALSE ("LBCB Number Button")) -> ()
            n77 = local write "LBCB Number"(LBCB_Number."LBCB1" ("LBCB Number")) -> ()
            n78 = Send Notification(notification=Update_Actions."Update", notifier=w208, error in (no error)=w207) -> (notifier out=w205:refnum<notifier>, error out=w206:errorcluster)
          }
          frame #1 {
          }
        }
        n79 = local write "Number of LBCBs"(w194) -> ()
        n80 = call "Number Of LBCBs DAO.vi"("Rigid Connection In"=w196, "Number of\nLBCBs In"=w194, "Actions"=Persistant_DAO_Actions."Set") -> ()  [unwired: 2 in, 7 out]
      }
      event #21 {
        w217 = FALSE ("Load")
        n81 = event-data() -> ()  [unwired: 4 out]
        n82 = local write "Load"(w217) -> ()
        n83 = local write "Save"(w217) -> ()
        n84 = property on="Save" class="Bool (strict)"() -> ("Blinking"=w216:bool)  [unwired: 2 in, 2 out]
        n85 = property on="Load" class="Bool (strict)"() -> ("Blinking"=w215:bool)  [unwired: 2 in, 2 out]
      }
      event #22 {
        n86 = event-data() -> ("NewVal"=w218:T3)  [unwired: 1 out]
        n87 = call "Actuator Disp Boundary DAO.vi"("error in (no error)"=w222, "Limit Boundary Parameters In"=w218, "Actions"=Persistant_DAO_Actions."Set") -> ("error out"=w221:errorcluster)  [unwired: 1 in, 7 out]
      }
      event #23 {
        n88 = event-data() -> ("NewVal"=w224:T3)  [unwired: 1 out]
        n89 = call "Actuator Force Boundary DAO.vi"("error in (no error)"=w228, "Limit Boundary Parameters In"=w224, "Actions"=Persistant_DAO_Actions."Set") -> ("error out"=w227:errorcluster)  [unwired: 1 in, 7 out]
      }
      event #24 {
        n90 = event-data() -> ("NewVal"=w230:T3)  [unwired: 1 out]
        n91 = call "Cartesian Moment Boundary DAO.vi"("error in (no error)"=w234, "Limit Boundary Parameters In"=w230, "Actions"=Persistant_DAO_Actions."Set") -> ("error out"=w233:errorcluster)  [unwired: 1 in, 7 out]
      }
      event #25 {
        n92 = event-data() -> ("NewVal"=w236:T3)  [unwired: 1 out]
        n93 = call "Cartesian Force Boundary DAO.vi"("error in (no error)"=w240, "Limit Boundary Parameters In"=w236, "Actions"=Persistant_DAO_Actions."Set") -> ("error out"=w239:errorcluster)  [unwired: 2 in, 6 out]
      }
      event #26 {
        n94 = event-data() -> ("NewVal"=w242:T3)  [unwired: 1 out]
        n95 = call "Cartesian Translation Boundary DAO.vi"("error in (no error)"=w246, "Limit Boundary Parameters In"=w242, "Actions"=Persistant_DAO_Actions."Set") -> ("error out"=w245:errorcluster)  [unwired: 1 in, 7 out]
      }
      event #27 {
        n96 = event-data() -> ("NewVal"=w248:T3)  [unwired: 1 out]
        n97 = call "Cartesian Rotation Boundary DAO.vi"("error in (no error)"=w252, "Limit Boundary Parameters In"=w248, "Actions"=Persistant_DAO_Actions."Set") -> ("error out"=w251:errorcluster)  [unwired: 1 in, 7 out]
      }
      event #28 {
        n98 = event-data() -> ("NewVal"=w255:T20)  [unwired: 1 out]
        n99 = call "Stiffness Jacobian DAO.vi"("error in (no error)"=w259, "Stiffness Jacobian In"=w255, "LBCB Number"=w254, "Actions"=Persistant_DAO_Actions."Set") -> ("error out"=w258:errorcluster)  [unwired: 1 in, 6 out]
      }
      event #29 {
        n100 = event-data() -> ("NewVal"=w261:T5)  [unwired: 6 out]
        n101 = call "LVDT Sensitivity DAO.vi"("error in (no error)"=w264, "LVDT Sensitivity Offset In"=w261, "LBCB Number"=w265, "Actions"=Persistant_DAO_Actions."Set") -> ("error out"=w263:errorcluster)  [unwired: 1 in, 6 out]
      }
      event #30 {
        n102 = event-data() -> ("NewVal"=w270:T5)  [unwired: 6 out]
        n103 = call "Command Sensitivity DAO.vi"("error in (no error)"=w273, "Command Sensitivity Offset In"=w270, "LBCB Number"=w271, "Actions"=Persistant_DAO_Actions."Set") -> ("error out"=w274:errorcluster)  [unwired: 1 in, 6 out]
      }
      event #31 {
        n104 = event-data() -> ("NewVal"=w277:T5)  [unwired: 6 out]
        n105 = call "Load Cell Sensitivity DAO.vi"("error in (no error)"=w279, "Load Cell Sensitivity Offset In"=w277, "LBCB Number"=w281, "Actions"=Persistant_DAO_Actions."Set") -> ("error out"=w278:errorcluster)  [unwired: 1 in, 6 out]
      }
      event #32 {
        n106 = event-data() -> ("NewVal"=w284:T5)  [unwired: 6 out]
        n107 = call "Load Cell Offsets DAO.vi"("error in (no error)"=w286, "Load Cell Displacement Offset In"=w284, "LBCB Number"=w288, "Actions"=Persistant_DAO_Actions."Set") -> ("error out"=w285:errorcluster)  [unwired: 1 in, 6 out]
      }
      event #33 {
        n108 = event-data() -> ("NewVal"=w289:T5)  [unwired: 1 out]
        n109 = call "LVDT Offsets DAO.vi"("error in (no error)"=w293, "LVDT Displacements Offset In"=w289, "LBCB Number"=w295, "Actions"=Persistant_DAO_Actions."Set") -> ("error out"=w292:errorcluster)  [unwired: 1 in, 6 out]
      }
      event #34 {
        w299 = Persistant_DAO_Actions."Set" ("Persistent DAO Actions")
        n110 = event-data() -> ("NewVal"=w298:T22[])  [unwired: 1 out]
        n111 = Empty Array?(array=w298) -> (empty?=w297:bool)
        n112 = case shown="True" w297 {
          tunnel: w298 -> [w308 _]
          tunnel: [w307 refnum<k21>[] []] -> w302
          tunnel: [w306 string[] []] -> w301
          tunnel: [w305 dbl[] []] -> w300
          frame #0 {
            n113 = for {
              tunnel: w308 -> [w312] mode=indexing
              tunnel: [w311] -> w307 mode=indexing
              tunnel: [w310] -> w306 mode=indexing
              tunnel: [w309] -> w305 mode=indexing
              n114 = Unbundle By Name(w312) -> ("DAQmx Global Channel"=w311:refnum<k21>, "Display Name"=w310:string, "Sensitivity"=w309:dbl)
            }
          }
          frame #1 {
          }
        }
        n115 = call "External Sensor Channel Names DAO.vi"("DAQ Channel In"=w302, "Persistent DAO Actions"=w299) -> ()  [unwired: 2 in, 8 out]
        n116 = call "External Sensor Display Names DAO.vi"("Display Name In"=w301, "Persistent DAO Actions"=w299) -> ()  [unwired: 2 in, 8 out]
        n117 = call "External Sensor Sensitivities DAO.vi"("Sensitivities In"=w300, "Persistent DAO Actions"=w299) -> ()  [unwired: 2 in, 8 out]
      }
      event #35 {
        n118 = event-data() -> ("NewVal"=w318:T21)  [unwired: 1 out]
        n119 = call "Command Channel Names DAO.vi"("error in (no error)"=w321, "Names In"=w318, "LBCB Number"=w319, "Actions"=Persistant_DAO_Actions."Set") -> ("error out"=w322:errorcluster)  [unwired: 1 in, 6 out]
      }
      event #36 {
        n120 = event-data() -> ("NewVal"=w323:T21)  [unwired: 1 out]
        n121 = call "LVDT Channel Names DAO.vi"("error in (no error)"=w328, "Names In"=w323, "LBCB Number"=w326, "Actions"=Persistant_DAO_Actions."Set") -> ("error out"=w329:errorcluster)  [unwired: 1 in, 6 out]
      }
      event #37 {
        n122 = event-data() -> ("NewVal"=w330:T21)  [unwired: 1 out]
        n123 = call "Load Cell Channel Names DAO.vi"("error in (no error)"=w335, "Names In"=w330, "LBCB Number"=w333, "Actions"=Persistant_DAO_Actions."Set") -> ("error out"=w336:errorcluster)  [unwired: 1 in, 6 out]
      }
      event #38 {
        n124 = event-data() -> ("NewVal"=w337:T21)  [unwired: 1 out]
        n125 = call "Servo Error Channel Names DAO.vi"("error in (no error)"=w342, "Names In"=w337, "LBCB Number"=w340, "Actions"=Persistant_DAO_Actions."Set") -> ("error out"=w343:errorcluster)  [unwired: 1 in, 6 out]
      }
      event #39 {
        n126 = event-data() -> ("NewVal"=w344:T5)  [unwired: 1 out]
        n127 = call "Servo Error Offset DAO.vi"("error in (no error)"=w349, "Servo Error Offset In"=w344, "LBCB Number"=w347, "Actions"=Persistant_DAO_Actions."Set") -> ("error out"=w350:errorcluster)  [unwired: 1 in, 6 out]
      }
      event #40 {
        n128 = event-data() -> ("NewVal"=w351:T17)  [unwired: 1 out]
        n129 = call "Default Ramp Time DAO.vi"("Ramp Time Actions"=Persistant_DAO_Actions."Set" ("Actions"), "Ramp Time In"=w351, "error in (no error)"=w355) -> ("error out"=w354:errorcluster)  [unwired: 2 in, 10 out]
      }
      event #41 {
        n130 = event-data() -> ("NewVal"=w357:T9)  [unwired: 1 out]
        n131 = call "DAQ Link Network Parameters DAO.vi"("error in (no error)"=w361, "Network Parameters In"=w357, "Persistent DAO Actions"=Persistant_DAO_Actions."Set" ("Actions")) -> ("error out"=w360:errorcluster)  [unwired: 6 in, 2 out]
      }
      event #42 {
        n132 = event-data() -> ("NewVal"=w363:T9)  [unwired: 1 out]
        n133 = call "NTCP Network Parameters DAO.vi"("error in (no error)"=w367, "Network Parameters In"=w363, "Persistent DAO Actions"=Persistant_DAO_Actions."Set" ("Actions")) -> ("error out"=w366:errorcluster)  [unwired: 6 in, 2 out]
      }
      event #43 {
        n134 = event-data() -> ("NewVal"=w370:T7)  [unwired: 1 out]
        n135 = call "Mixed Mode Force Group Priorities DAO.vi"("Force Error Range Actions"=Persistant_DAO_Actions."Set" ("Actions"), "Force Group Priorities In"=w370, "LBCB Number"=w374, "error in (no error)"=w373) -> ("error out"=w372:errorcluster)  [unwired: 9 in, 2 out]
      }
      event #44 {
        n136 = event-data() -> ("NewVal"=w376:T6)  [unwired: 1 out]
        n137 = call "Stiffness Limits DAO.vi"("Cartesian Force Limit Actions"=Persistant_DAO_Actions."Set" ("Actions"), "ID"=w381, "Stiffness Limit In"=w376, "error in (no error)"=w380) -> ("error out"=w379:errorcluster)  [unwired: 9 in, 2 out]
      }
      event #45 {
        n138 = event-data() -> ("NewVal"=w383:T16)  [unwired: 1 out]
        n139 = call "Force Control Parameters DAO.vi"("error in (no error)"=w387, "Force Control Parameters In"=w383, "DAO Actions"=Persistant_DAO_Actions."Set" ("Actions")) -> ("error out"=w386:errorcluster)  [unwired: 6 in, 2 out]
      }
      event #46 {
        n140 = event-data() -> ("NewVal"=w391:bool)  [unwired: 1 out]
        n141 = local read "Number of LBCBs"() -> (w389:T1)
        n142 = case shown="True" w391 {
          tunnel: w397 -> [w400 w406]
          tunnel: w396 -> [w399 w405]
          tunnel: [w399 w404] -> w395
          tunnel: [w400 w403] -> w394
          tunnel: [w398 Number_Of_LBCBs."2" ("Number of LBCBs")] -> w390
          tunnel: w389 -> [w398 _]
          frame #0 {
          }
          frame #1 {
            n143 = Send Notification(notification=Update_Actions."Update", notifier=w406, error in (no error)=w405) -> (notifier out=w403:refnum<notifier>, error out=w404:errorcluster)
          }
        }
        n144 = local write "Number of LBCBs"(w390) -> ()
        n145 = call "Number Of LBCBs DAO.vi"("Rigid Connection In"=w391, "Number of\nLBCBs In"=w390, "Actions"=Persistant_DAO_Actions."Set") -> ()  [unwired: 2 in, 7 out]
      }
      event #47 {
        n146 = event-data() -> ("NewVal"=w407:T2)  [unwired: 1 out]
        n147 = local read "Number of LBCBs"() -> (w410:T1)
        n148 = local read "Rigid Connection"() -> (w409:bool)
        n149 = call "OM Setup Page Filter.vi"("OM Setup Page"=w407, "Rigid Connection In"=w409, "Number of\nLBCBs In"=w410, "LBCB Number In"=w408) -> ("LBCB Number Out"=w411:T24)  [unwired: 7 in]
        n150 = local write "LBCB Number"(w411) -> ()
        n151 = Send Notification(notification=Update_Actions."Update", notifier=w415, error in (no error)=w417) -> (notifier out=w414:refnum<notifier>, error out=w416:errorcluster)
      }
    }
    n152 = call "Error Logger.vi"("error in (no error)"=w22) -> ("error out"=w21:errorcluster)  [unwired: 1 in, 9 out]
    n153 = property on="Load" class="Bool (strict)"("Blinking"=w16) -> ()  [unwired: 2 in, 2 out]
    n154 = property on="Save" class="Bool (strict)"("Blinking"=w17) -> ()  [unwired: 2 in, 2 out]
  }
  n155 = while {
    shift-right: [w421] -> _
    shift-left: w9 -> [w424]
    tunnel: w8 -> [w419]
    tunnel: [w418] -> w3
    stop <- w418 stop-if-true
    # "Monitor Loop"
    n156 = Wait on Notification(notifier=w424, timeout in ms (-1)=2000, error in (no error)=w419) -> (notifier out=w421:refnum<notifier>, notification=w420:T25, timed out?=w422:bool)  [unwired: 2 out]
    n157 = case shown="False" w422 {
      tunnel: w420 -> [w426 _]
      tunnel: [w425 _] -> w418
      frame #0 {
        n158 = case shown="\"Update\"" w426 {
          tunnel: [_ TRUE] -> w425
          frame #0 {
            w432 = Persistant_DAO_Actions."Get" ("Actions")
            n159 = local read "LBCB Number"() -> (w431:T24)
            n160 = call "LBCB Position DAO.vi"("LBCB Settings Actions"=w432, "LBCB Number"=w431) -> ("LBCB Position Output"=w472:T12)  [unwired: 3 in, 10 out]
            n161 = call "OM Location Dao.vi"("Actions"=w432) -> ("LBCB  Location Out"=w473:T23)  [unwired: 3 in, 7 out]
            n162 = call "Number Of LBCBs DAO.vi"("Actions"=w432) -> ("Rigid Connection Out"=w427:bool, "Number of\nLBCBs Out"=w470:T1)  [unwired: 4 in, 5 out]
            n163 = call "Actuator Force Limit DAO.vi"("Actuator Force Limit Actions"=w432, "ID"=w431) -> ("Actuator Force Limits Out"=w466:T4)  [unwired: 3 in, 10 out]
            n164 = call "Actuator Stroke Limit DAO.vi"("Actuator Stroke Limit Actions"=w432, "ID"=w431) -> ("Actuator Stroke Limits Out"=w467:T4)  [unwired: 3 in, 10 out]
            n165 = call "Command Voltage Limit DAO.vi"("Actuator Stroke Limit Actions"=w432, "ID"=w431) -> ("Command Voltage Limit Out"=w465:T4)  [unwired: 3 in, 10 out]
            n166 = call "App Parameters DAO.vi"("Actions"=w432) -> ("Application Timing and Logging Out"=w464:T10)  [unwired: 3 in, 7 out]
            n167 = call "LVDT Sensitivity DAO.vi"("LBCB Number"=w431, "Actions"=w432) -> ("LVDT Sensitivity Offsets Out"=w450:T5)  [unwired: 3 in, 6 out]
            n168 = call "Stiffness Limits DAO.vi"("Cartesian Force Limit Actions"=w432, "ID"=w431) -> ("Stiffness Limit Out"=w430:T6)  [unwired: 11 in, 2 out]
            n169 = call "Mixed Mode Force Group Priorities DAO.vi"("Force Error Range Actions"=w432, "LBCB Number"=w431) -> ("Force Group Priorities Out"=w429:T7)  [unwired: 11 in, 2 out]
            n170 = call "Force Control Parameters DAO.vi"("DAO Actions"=w432) -> ("Force Control Parameters Out"=w428:T16)  [unwired: 8 in, 2 out]
            n171 = call "Load Cell Sensitivity DAO.vi"("LBCB Number"=w431, "Actions"=w432) -> ("Load Cell Sensitivity Offsets Out"=w449:T5)  [unwired: 3 in, 6 out]
            n172 = local write "Application Timing and Logging"(w464) -> ()
            n173 = local write "Load Cell Sensitivity"(w449) -> ()
            n174 = local write "Command Voltage Limit"(w465) -> ()
            n175 = local write "Actuator Stroke Limits"(w467) -> ()
            n176 = local write "LVDT Sensitivity"(w450) -> ()
            n177 = local write "Actuator Force Limits"(w466) -> ()
            n178 = local write "Rigid Connection"(w427) -> ()
            n179 = local write "Number of LBCBs"(w470) -> ()
            n180 = local write "LBCB Position"(w472) -> ()
            n181 = local write "OM  Location"(w473) -> ()
            n182 = local write "Force Control Parameters"(w428) -> ()
            n183 = local write "Force Group Priorities"(w429) -> ()
            n184 = local write "Stiffness Limit"(w430) -> ()
            n185 = call "LBCB Settings DAO.vi"("LBCB Number"=w431, "Actions"=w432) -> ("LBCB Setting Out"=w471:T13)  [unwired: 3 in, 6 out]
            n186 = call "Cartesian Force Limit DAO.vi"("Cartesian Force Limit Actions"=w432, "ID"=w431) -> ("Cartesian Force Limit Out"=w468:T6)  [unwired: 3 in, 10 out]
            n187 = call "Cartesian Displacement Limit DAO.vi"("Cartesian Displacement Limit Actions"=w432, "ID"=w431) -> ("Cartesian Displacement Out"=w469:T6)  [unwired: 3 in, 10 out]
            n188 = call "Autobalance Control DAO.vi"("Persistent DAO Actions"=w432) -> ("Autobalance Control Out"=w441:T8)  [unwired: 3 in, 7 out]
            n189 = call "Auto Balance Error Tolerance DAO.vi"("Auto Balance Increment Actions"=w432, "LBCB Number"=w431) -> ("Auto Balance Error Out"=w463:T5)  [unwired: 3 in, 10 out]
            n190 = call "NTCP Network Parameters DAO.vi"("Persistent DAO Actions"=w432) -> ("Network Parameters Out"=w433:T9)  [unwired: 8 in, 2 out]
            n191 = call "Command Sensitivity DAO.vi"("LBCB Number"=w431, "Actions"=w432) -> ("Command Sensitivity Offsets Out"=w446:T5)  [unwired: 3 in, 6 out]
            n192 = call "LVDT Offsets DAO.vi"("LBCB Number"=w431, "Actions"=w432) -> ("LVDT Displacements Offsets Out"=w448:T5)  [unwired: 3 in, 6 out]
            n193 = call "DAQ Link Network Parameters DAO.vi"("Persistent DAO Actions"=w432) -> ("Network Parameters Out"=w434:T9)  [unwired: 8 in, 2 out]
            n194 = local write "Cartesian Displacement"(w469) -> ()
            n195 = local write "Auto Balance Error Window"(w463) -> ()
            n196 = local write "Auto Balance Control"(w441) -> ()
            n197 = local write "Cartesian Force Limit"(w468) -> ()
            n198 = local write "NTCP Network"(w433) -> ()
            n199 = local write "DAQ Link Network"(w434) -> ()
            n200 = local write "LBCB Settings"(w471) -> ()
            n201 = local write "Command Sensitivity"(w446) -> ()
            n202 = local write "LVDT  Offset"(w448) -> ()
            n203 = call "Mixed Mode Force Error Range DAO.vi"("Force Error Range Actions"=w432, "LBCB Number"=w431) -> ("Force Error Range Out"=w462:T7)  [unwired: 3 in, 10 out]
            n204 = call "Mixed Mode Jacobian Gain DAO.vi"("Jacobian Gain Actions"=w432, "LBCB Number"=w431) -> ("Jacobian Gain Out"=w461:T7)  [unwired: 3 in, 10 out]
            n205 = call "Stiffness Jacobian DAO.vi"("LBCB Number"=w431, "Actions"=w432) -> ("Stiffness Jacobian Out"=w460:T20)  [unwired: 3 in, 6 out]
            n206 = call "Mixed Mode Max Increment DAO.vi"("Max Increment Actions"=w432, "LBCB Number"=w431) -> ("Max Increment Out"=w459:T7)  [unwired: 3 in, 10 out]
            n207 = call "P Gain DAO.vi"("P Gain Actions"=w432, "LBCB Number"=w431) -> ("P Gain"=w458:T5)  [unwired: 3 in, 10 out]
            n208 = call "I Gain DAO.vi"("I Gain Actions"=w432, "LBCB Number"=w431) -> ("I Gain"=w457:T5)  [unwired: 3 in, 10 out]
            n209 = call "Load Cell Offsets DAO.vi"("LBCB Number"=w431, "Actions"=w432) -> ("Load Cell Displacement Offsets Out"=w447:T5)  [unwired: 3 in, 6 out]
            n210 = call "Default Ramp Time DAO.vi"("Ramp Time Actions"=w432) -> ("Ramp Time Out"=w435:T17)  [unwired: 3 in, 11 out]
            n211 = local write "Stiffness Jacobian"(w460) -> ()
            n212 = local write "Force Error Range"(w462) -> ()
            n213 = local write "Max Increment"(w459) -> ()
            n214 = local write "Jacobian Gain"(w461) -> ()
            n215 = local write "Default Ramp Times"(w435) -> ()
            n216 = local write "Load Cell  Offset"(w447) -> ()
            n217 = local write "P Gain"(w458) -> ()
            n218 = local write "I Gain"(w457) -> ()
            n219 = call "Actuator Disp Boundary DAO.vi"("Actions"=w432) -> ("Limit Boundary Parameters Out"=w456:T3)  [unwired: 3 in, 7 out]
            n220 = call "Actuator Force Boundary DAO.vi"("Actions"=w432) -> ("Limit Boundary Parameters Out"=w455:T3)  [unwired: 3 in, 7 out]
            n221 = call "Cartesian Moment Boundary DAO.vi"("Actions"=w432) -> ("Limit Boundary Parameters Out"=w454:T3)  [unwired: 3 in, 7 out]
            n222 = call "Cartesian Force Boundary DAO.vi"("Actions"=w432) -> ("Limit Boundary Parameters Out"=w453:T3)  [unwired: 3 in, 7 out]
            n223 = call "Cartesian Translation Boundary DAO.vi"("Actions"=w432) -> ("Limit Boundary Parameters Out"=w452:T3)  [unwired: 3 in, 7 out]
            n224 = call "Cartesian Rotation Boundary DAO.vi"("Actions"=w432) -> ("Limit Boundary Parameters Out"=w451:T3)  [unwired: 3 in, 7 out]
            n225 = call "External Sensor Channel Names DAO.vi"("Persistent DAO Actions"=w432) -> ("DAQ Channel Out"=w445:refnum<k21>[])  [unwired: 3 in, 7 out]
            n226 = call "External Sensor Display Names DAO.vi"("Persistent DAO Actions"=w432) -> ("Display Name Out"=w444:string[])  [unwired: 3 in, 7 out]
            n227 = call "External Sensor Sensitivities DAO.vi"("Persistent DAO Actions"=w432) -> ("Sensitivities Out"=w443:dbl[])  [unwired: 3 in, 7 out]
            n228 = local write "Cart Trans Bnd"(w452) -> ()
            n229 = local write "Cart Mmt Bnd"(w454) -> ()
            n230 = local write "Cart Rot Bnd"(w451) -> ()
            n231 = local write "Cart Force Bnd"(w453) -> ()
            n232 = local write "Act Force Bnd"(w455) -> ()
            n233 = local write "Act Disp Bnd"(w456) -> ()
            n234 = for {
              tunnel: w445 -> [w477] mode=indexing
              tunnel: w444 -> [w476] mode=indexing
              tunnel: w443 -> [w475] mode=indexing
              tunnel: [w474] -> w442 mode=indexing
              n235 = Bundle By Name(cluster=T22 {"DAQmx Global Channel"="", "Display Name"="", "Sensitivity"=0.0} ("External Sensor Spec"), "DAQmx Global Channel"=w477, "Display Name"=w476, "Sensitivity"=w475) -> (w474:T22)
            }
            n236 = call "Servo Error Offset DAO.vi"("LBCB Number"=w431, "Actions"=w432) -> ("Servo Error  Offsets Out"=w436:T5)  [unwired: 3 in, 6 out]
            n237 = call "Command Channel Names DAO.vi"("LBCB Number"=w431, "Actions"=w432) -> ("Names Out"=w440:T21)  [unwired: 3 in, 6 out]
            n238 = call "LVDT Channel Names DAO.vi"("LBCB Number"=w431, "Actions"=w432) -> ("Names Out"=w439:T21)  [unwired: 3 in, 6 out]
            n239 = call "Load Cell Channel Names DAO.vi"("LBCB Number"=w431, "Actions"=w432) -> ("Names Out"=w438:T21)  [unwired: 3 in, 6 out]
            n240 = call "Servo Error Channel Names DAO.vi"("LBCB Number"=w431, "Actions"=w432) -> ("Names Out"=w437:T21)  [unwired: 3 in, 6 out]
            n241 = local write "Command Channels"(w440) -> ()
            n242 = local write "LVDT Channels"(w439) -> ()
            n243 = local write "Load Cell Channels"(w438) -> ()
            n244 = local write "External Sensor Specs"(w442) -> ()
            n245 = local write "Servo Error  Channels"(w437) -> ()
            n246 = local write "Servo Error Offset"(w436) -> ()
          }
          frame #1 {
          }
        }
      }
      frame #1 {
      }
    }
  }
  n247 = Compound Arithmetic op=AND(w4, w3) -> (w2:bool)
  n248 = Not(x=w2) -> (.not. x?=w1:bool)
  n249 = flat-sequence {
    tunnel: w1 -> [w481]
    frame #0 {
      n250 = control-ref of="This VI"() -> (w480:refnum<vi>)
      n251 = invoke class="VI" method="FP.Close"(reference=w480) -> ()  [unwired: 2 in, 3 out]
      n252 = local write "Ok"(w481) -> ()
    }
  }
